vi "(SubVI)_Control_CreateFile_MultiSite_ver17.vi"(9 "Control tab Label":string, 10 "Control Tab\nParameters":T1, 11 "Path":path=path "C:/OCT_Data") -> (0 "error out":errorcluster, 2 "Controller_Data_File":refnum<file>, 3 "Doppler_Data_File":refnum<file>)   [LabVIEW 2019]
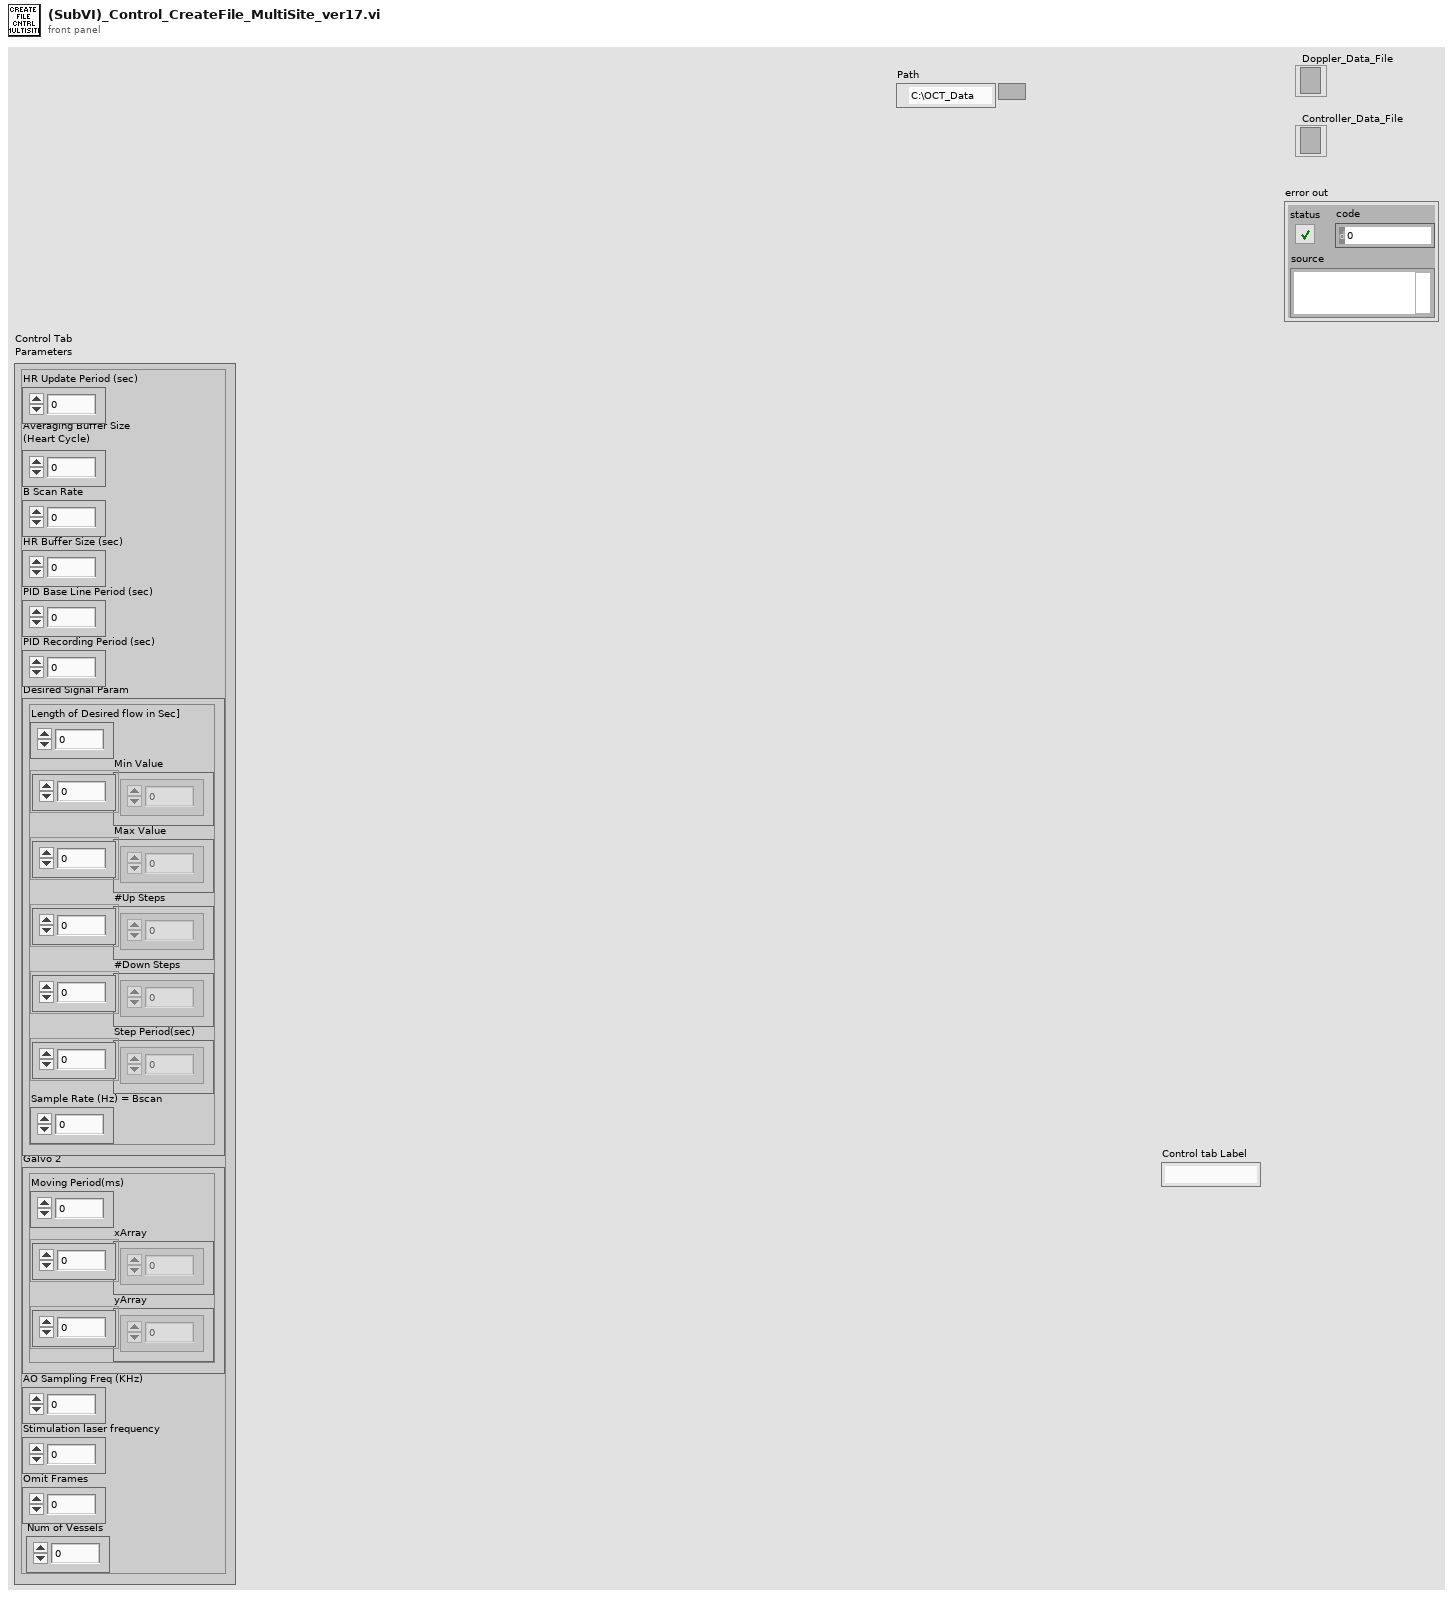
[diagram p1: front panel]
types:
  T1 = cluster{"HR Update Period (sec)":i32, "Averaging Buffer Size\n(Heart Cycle)":dbl, "B Scan Rate":dbl, "HR Buffer Size (sec)":dbl, "PID Base Line Period (sec) ":dbl, "PID Recording Period (sec) ":dbl, "Desired Signal Param":cluster{"Length of Desired flow in Sec]":dbl, "Min Value":dbl[], "Max Value":dbl[], "#Up Steps":dbl[], "#Down Steps":dbl[], "Step Period(sec)":dbl[], "Sample Rate (Hz) = Bscan":dbl}, "Galvo 2":cluster{"Moving Period(ms)":dbl, "xArray":dbl[], "yArray":dbl[]}, "AO Sampling Freq (KHz)":dbl, "Stimulation laser frequency":dbl, "Omit Frames":i32, "Num of Vessels":i32}
  T2 = enum16{"big-endian, network order", "native, host order", "little-endian"}
  T3 = enum16{"open", "replace", "create", "open or create", "replace or create", "replace or create with confirmation"}
  T4 = cluster{"Length of Desired flow in Sec]":dbl, "Min Value":dbl[], "Max Value":dbl[], "#Up Steps":dbl[], "#Down Steps":dbl[], "Step Period(sec)":dbl[], "Sample Rate (Hz) = Bscan":dbl}
  T5 = cluster{"Moving Period(ms)":dbl, "xArray":dbl[], "yArray":dbl[]}
  T6 = cluster{"string":string, dbl, "string":string, "Averaging Buffer Size\n(Heart Cycle)":dbl, "string":string, "B Scan Rate":dbl, "string":string, "HR Buffer Size (sec)":dbl}
  T7 = cluster{"string":string, "PID Base Line Period (sec) ":dbl, "string":string, "PID Recording Period (sec) ":dbl}
  T8 = cluster{"string":string, dbl[], "string":string, dbl[], "string":string, "Step Period(sec)":dbl[], "string":string, "Min Value":dbl[], "string":string, "Max Value":dbl[], "string":string, "Sample Rate (Hz) = Bscan":dbl}
  T9 = cluster{"string":string, "string":string, "string":string, "Scan Angle 2D":dbl}
  T10 = cluster{"string":string, "Moving Period(ms)":dbl, "string":string, dbl, "string":string, "xArray":dbl[], "string":string, dbl, "string":string, "yArray":dbl[], "string":string, "AO Sampling Freq (KHz)":dbl, "string":string, "Stimulation laser frequency":dbl, "string":string, dbl, "string":string, dbl}
  T11 = cluster{"string":string, "string":string, "string":string, "string":string}
  T12 = cluster{cluster{"string":string, "string":string, "string":string, "Scan Angle 2D":dbl}, cluster{"string":string, dbl, "string":string, "Averaging Buffer Size\n(Heart Cycle)":dbl, "string":string, "B Scan Rate":dbl, "string":string, "HR Buffer Size (sec)":dbl}, cluster{"string":string, "PID Base Line Period (sec) ":dbl, "string":string, "PID Recording Period (sec) ":dbl}, cluster{"string":string, dbl[], "string":string, dbl[], "string":string, "Step Period(sec)":dbl[], "string":string, "Min Value":dbl[], "string":string, "Max Value":dbl[], "string":string, "Sample Rate (Hz) = Bscan":dbl}, cluster{"string":string, "Moving Period(ms)":dbl, "string":string, dbl, "string":string, "xArray":dbl[], "string":string, dbl, "string":string, "yArray":dbl[], "string":string, "AO Sampling Freq (KHz)":dbl, "string":string, "Stimulation laser frequency":dbl, "string":string, dbl, "string":string, dbl}, "string":string, "string":string}
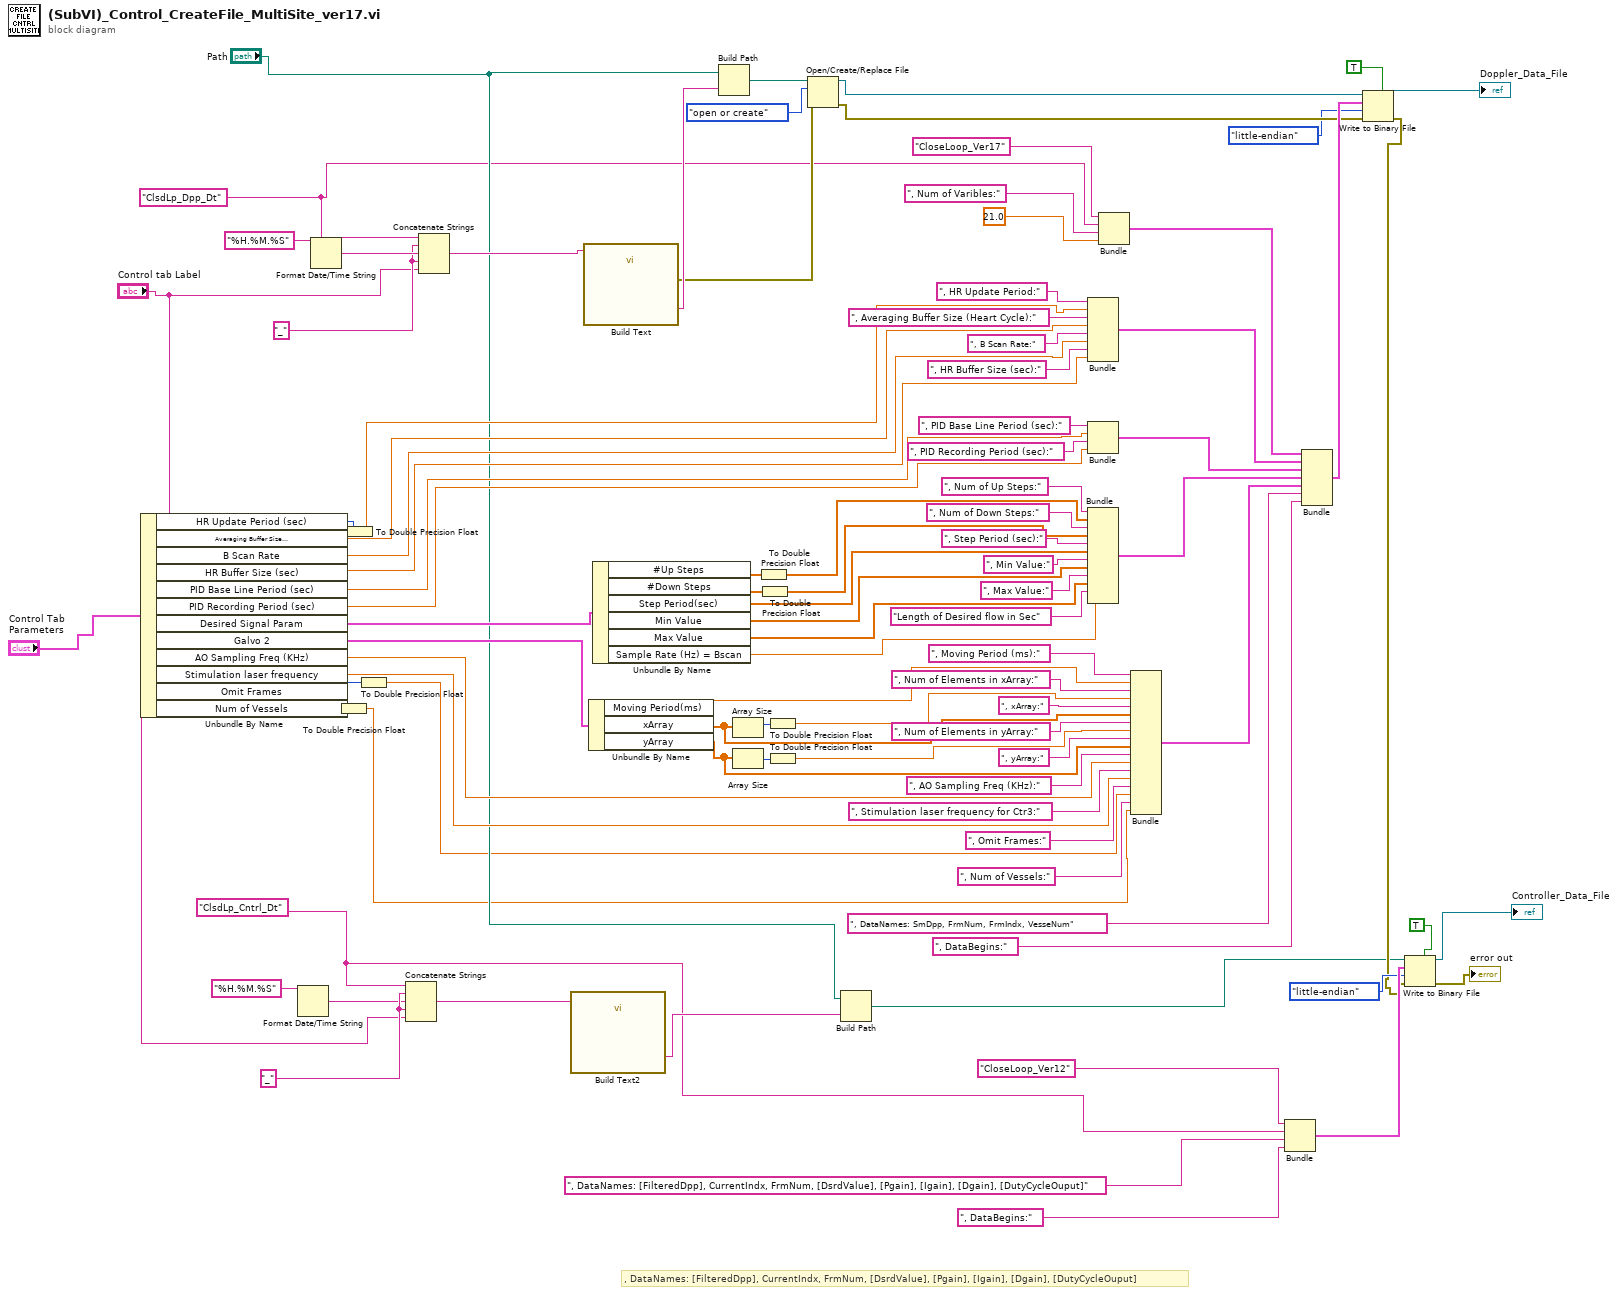
[diagram p0: block diagram]
diagram:
  w9 = "ClsdLp_Cntrl_Dt" ("string")
  w10 = "ClsdLp_Dpp_Dt" ("string")
  w30 = "_" ("3D Label")
  w91 = "_" ("3D Label")
  # ", DataNames: [FilteredDpp], CurrentIndx, FrmNum, [DsrdValue], [Pgain], [Igain], [Dgain], [DutyCycleOuput]"
  n1 = Unbundle By Name("Control Tab\nParameters") -> ("HR Update Period (sec)"=w74:i32, "Averaging Buffer Size\n(Heart Cycle)"=w56:dbl, "B Scan Rate"=w55:dbl, "HR Buffer Size (sec)"=w54:dbl, "PID Base Line Period (sec)"=w53:dbl, "PID Recording Period (sec)"=w52:dbl, "Desired Signal Param"=w78:T4, "Galvo 2"=w77:T5, "AO Sampling Freq (KHz)"=w37:dbl, "Stimulation laser frequency"=w36:dbl, "Omit Frames"=w7:i32, "Num of Vessels"=w3:i32)
  n2 = Format Date/Time String(time format string (%c)="%H.%M.%S") -> (date/time string=w28:string)  [unwired: 2 in]
  n3 = Format Date/Time String(time format string (%c)="%H.%M.%S") -> (date/time string=w94:string)  [unwired: 2 in]
  n4 = To Double Precision Float(number=w3) -> (double precision float=w2:dbl)
  n5 = To Double Precision Float(number=w74) -> (double precision float=w57:dbl)
  n6 = To Double Precision Float(number=w7) -> (double precision float=w6:dbl)
  n7 = Concatenate Strings(w9, w30, w28, w30, "Control tab Label") -> (w29:string)
  n8 = Concatenate Strings(w10, w91, w94, w91, "Control tab Label") -> (w93:string)
  n9 = call "Build Text2"("Beginning Text"=w29) -> ("Result"=w13:string)  [unwired: 13 in, 1 out]
  n10 = call "Build Text"("Beginning Text"=w93) -> ("Result"=w92:string, "error out"=w25:errorcluster)  [unwired: 13 in]
  n11 = Unbundle By Name(w77) -> ("Moving Period(ms)"=w45:dbl, "xArray"=w41:dbl[], "yArray"=w39:dbl[])
  n12 = Unbundle By Name(w78) -> ("#Up Steps"=w75:dbl[], "#Down Steps"=w76:dbl[], "Step Period(sec)"=w49:dbl[], "Min Value"=w48:dbl[], "Max Value"=w47:dbl[], "Sample Rate (Hz) = Bscan"=w46:dbl)
  n13 = Build Path(base path="Path", name or relative path=w92) -> (appended path=w90:path)
  n14 = Array Size(array=w41) -> (size(s)=w44:i32)
  n15 = Array Size(array=w39) -> (size(s)=w43:i32)
  n16 = To Double Precision Float(number=w75) -> (double precision float=w50:dbl[])
  n17 = To Double Precision Float(number=w76) -> (double precision float=w5:dbl[])
  n18 = To Double Precision Float(number=w44) -> (double precision float=w42:dbl)
  n19 = To Double Precision Float(number=w43) -> (double precision float=w40:dbl)
  n20 = Open/Create/Replace File(file path (use dialog)=w90, error in=w25, operation (0:open)=T3."open or create") -> (refnum out=w86:refnum<file>, error out=w85:errorcluster)  [unwired: 3 in, 1 out]
  n21 = Build Path(base path="Path", name or relative path=w13) -> (appended path=w11:path)
  n22 = Bundle("string"=", HR Update Period:", w57, "string"=", Averaging Buffer Size (Heart Cycle):", "Averaging Buffer Size\n(Heart Cycle)"=w56, "string"=", B Scan Rate:", "B Scan Rate"=w55, "string"=", HR Buffer Size (sec):", "HR Buffer Size (sec)"=w54) -> (w34:T6)  [unwired: 1 in]
  n23 = Bundle("string"=", PID Base Line Period (sec):", "PID Base Line Period (sec)"=w53, "string"=", PID Recording Period (sec):", "PID Recording Period (sec)"=w52) -> (w33:T7)  [unwired: 1 in]
  n24 = Bundle("string"=", Num of Up Steps:", w50, "string"=", Num of Down Steps:", w5, "string"=", Step Period (sec):", "Step Period(sec)"=w49, "string"=", Min Value:", "Min Value"=w48, "string"=", Max Value:", "Max Value"=w47, "string"="Length of Desired flow in Sec", "Sample Rate (Hz) = Bscan"=w46) -> (w32:T8)  [unwired: 1 in]
  n25 = Bundle("string"="CloseLoop_Ver17", "string"=w10, "string"=", Num of Varibles:", "Scan Angle 2D"=21.0) -> (w88:T9)  [unwired: 1 in]
  n26 = Bundle("string"=", Moving Period (ms):", "Moving Period(ms)"=w45, "string"=", Num of Elements in xArray:", w42, "string"=", xArray:", "xArray"=w41, "string"=", Num of Elements in yArray:", w40, "string"=", yArray:", "yArray"=w39, "string"=", AO Sampling Freq (KHz):", "AO Sampling Freq (KHz)"=w37, "string"=", Stimulation laser frequency for Ctr3:", "Stimulation laser frequency"=w36, "string"=", Omit Frames:", w6, "string"=", Num of Vessels:", w2) -> (w31:T10)  [unwired: 1 in]
  n27 = Bundle("string"="CloseLoop_Ver12", "string"=w9, "string"=", DataNames: [FilteredDpp], CurrentIndx, FrmNum, [DsrdValue], [Pgain], [Igain], [Dgain], [DutyCycleOuput]", "string"=", DataBegins:") -> (w23:T11)  [unwired: 1 in]
  n28 = Bundle(w88, w34, w33, w32, w31, "string"=", DataNames: SmDpp, FrmNum, FrmIndx, VesseNum", "string"=", DataBegins:") -> (w87:T12)  [unwired: 1 in]
  n29 = Write to Binary File(file (use dialog)=w86, data=w87, error in=w85, 5:TRUE ("prepend array or string size? (T)"), 9:T2."little-endian" ("byte order (0:big-endian, network order)")) -> (refnum out=→"Doppler_Data_File":refnum<file>, error out=w20:errorcluster)  [unwired: 1 in, 1 out]
  n30 = Write to Binary File(file (use dialog)=w11, data=w23, error in=w20, 5:TRUE ("prepend array or string size? (T)"), 9:T2."little-endian" ("byte order (0:big-endian, network order)")) -> (refnum out=→"Controller_Data_File":refnum<file>, error out=→"error out":errorcluster)  [unwired: 1 in, 1 out]
